vi "MLS ident.vi"() -> ()   [LabVIEW 2015]
uses:
  <vilib>/FPGAPlugInAG/myRIO-1900/niLvFpga_Open_myRIO-1900.vi
  <vilib>/rvi/interface/common/dynamic/niFpgaDynamicAddResources.vi
  <vilib>/Utility/file.llb/Write Delimited Spreadsheet (I64).vi
  <vilib>/Utility/file.llb/Write Delimited Spreadsheet (DBL).vi
  <vilib>/Utility/error.llb/Error Cluster From Error Code.vi
  <vilib>/rvi/errors/niLvFpgaAdjustHostInterfaceError.vi
  <vilib>/FPGAPlugInAG/Dynamic/niLvFpga_Close_Dynamic.vi
  <vilib>/rvi/interface/nirviOpenFPGA/nirviOpenFPGA.xnode
  FPGA Bitfiles/ACC20115_FPGATarget_CurrentControlle_Dt5vFgOzYtY.lvbitx
  Current Controller.vi
  <vilib>/rvi/interface/nirviReadWriteControl/nirviReadWriteControl.xnode
  <vilib>/rvi/interface/nirviCloseFPGA/nirviCloseFPGA.xnode
  <vilib>/Analysis/NI_AALBase.lvlib
  NiFpgaLv.dll
  <vilib>/rvi/interface/Simulation/niFpgaSimulationCallBeginRW.vi
panel:
  out "error out":errorcluster
  in  "Stop":bool
  in  "Tab Control":enum32{"Monitor"}(tab)
  out "MLS":dbl[](graph)
  out "Sensor":dbl(graph)
  out "FPGA Status":bool
  out "Uniform White Noise":dbl[](graph)
  out "ms":u32
  in  "samples":i64=1
  out "Sampling Frequency":dbl(graph)
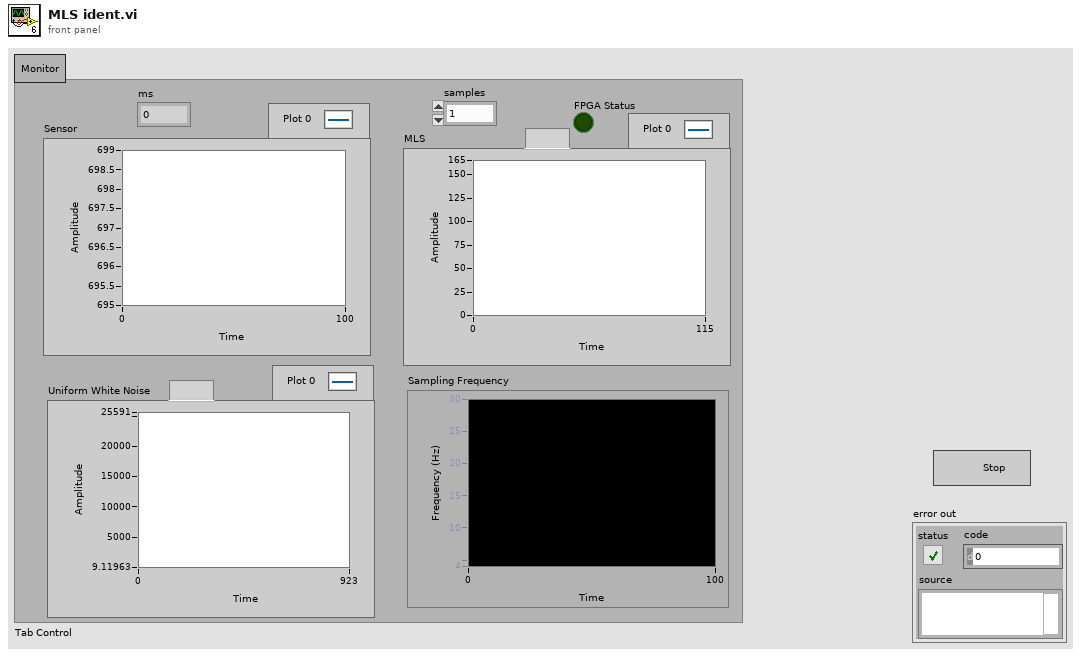
[diagram p1: front panel]
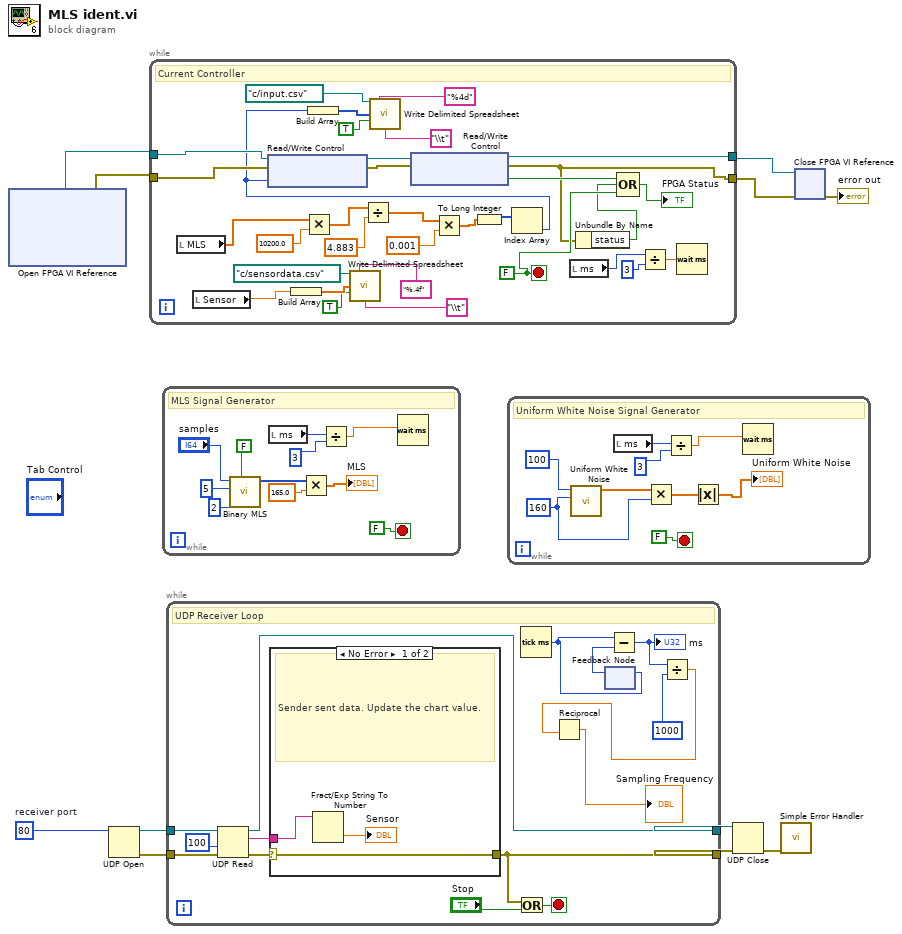
[diagram p0: block diagram]
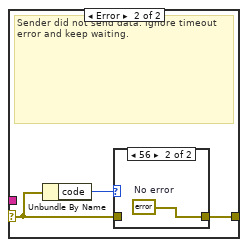
[diagram p2: hidden frame]
diagram:
  w2 = u16 80  # receiver port
  n1 = xnode "Open FPGA VI Reference"() -> ("FPGA VI Reference Out"=w11:refnum<k20>, "error out"=w10:errorcluster)  [unwired: 2 in]
  n2 = UDP Open(11:w2) -> (port=w3:refnum<k16>, 0:w4:errorcluster)  [unwired: 4 in, 1 out]
  n3 = while {
    tunnel: w11 -> [w44]
    tunnel: w10 -> [w43]
    tunnel: [w33] -> w9
    tunnel: [w29] -> w8
    stop <- w32 stop-if-true
    w32 = FALSE
    # "Current Controller"
    n4 = local read "MLS"() -> (w38:dbl[])
    n5 = local read "Sensor"() -> (w16:dbl)
    n6 = Build Array(w16) -> (w17:dbl[])
    n7 = Multiply(x=w38, y=10200.0) -> (x*y=w39:dbl[])
    n8 = call-poly <vilib>:"Write Delimited Spreadsheet.vi"("file path (dialog if empty)"=path "c:/sensordata.csv", "format (%.3f)"="%.4f", "1D data"=w17, "append to file? (F)"=TRUE, "delimiter (\\t)"="\\t" ("delimiter (\\t)")) -> ()  [unwired: 9 in, 2 out]
    n9 = Divide(x=w39, y=4.883) -> (x/y=w41:dbl[])
    n10 = Multiply(x=w41, y=0.001) -> (x*y=w37:dbl[])
    n11 = To Long Integer(number=w37) -> (32bit integer=w24:i32[])
    n12 = Index Array(array=w24) -> (element=w23:i32)  [unwired: 1 in]
    n13 = xnode "Read/Write Control"("FPGA VI Reference In"=w44, "error in"=w43, "DAC Inlet Valve"=w23) -> ("FPGA VI Reference Out"=w35:refnum<k20>, "error out"=w34:errorcluster)
    n14 = Build Array(w23) -> (w22:i32[])
    n15 = call-poly <vilib>:"Write Delimited Spreadsheet.vi"("file path (dialog if empty)"=path "c:/input.csv", "format (%d)"="%4d", "1D data"=w22, "append to file? (F)"=TRUE, "delimiter (\\t)"="\\t" ("delimiter (\\t)")) -> ()  [unwired: 9 in, 2 out]
    n16 = xnode "Read/Write Control"("FPGA VI Reference In"=w35, "error in"=w34) -> ("FPGA VI Reference Out"=w33:refnum<k20>, "error out"=w29:errorcluster, "Inlet Overflow?"=w30:bool)
    n17 = local read "ms"() -> (w28:u32)
    n18 = Unbundle By Name(w29) -> ("status"=w31:bool)
    n19 = Compound Arithmetic op=OR(w30, w31, w32) -> (→"FPGA Status":bool)
    n20 = Divide(x=w28, y=u32 3) -> (x/y=w26:dbl)
    n21 = Wait (ms)(milliseconds to wait=w26) -> ()  [unwired: 1 out]
  }
  n22 = while {
    stop <- FALSE stop-if-true
    # "MLS Signal Generator"
    n23 = call <vilib>:"Binary MLS.vi"("initialize?"=FALSE, "seed"=i64 2, "polynomial order"=5, "samples"="samples") -> ("mls sequence"=w52:u8[])  [unwired: 6 in, 1 out]
    n24 = local read "ms"() -> (w50:u32)
    n25 = Multiply(x=w52, y=165.0 ("amplitude")) -> (x*y=→"MLS":dbl[])
    n26 = Divide(x=w50, y=u32 3) -> (x/y=w48:dbl)
    n27 = Wait (ms)(milliseconds to wait=w48) -> ()  [unwired: 1 out]
  }
  n28 = while {
    tunnel: w3 -> [w70]
    tunnel: [w62] -> w7
    tunnel: w4 -> [w67]
    tunnel: [w63] -> w5
    stop <- w68 stop-if-true
    # "UDP Receiver Loop"
    n29 = UDP Read(connection ID=w70, timeout ms (25000)=100, 8:w67) -> (data out=w65:string, error out=w64:errorcluster, 3:w62:refnum<k16>)  [unwired: 3 out]
    n30 = case shown="No Error" w64 {
      selector: w64 -> [w71 w75]
      tunnel: w65 -> [w73 _]
      tunnel: [w71 w74] -> w63
      frame No Error {
        # "Sender sent data. Update the chart value."
        n31 = Fract/Exp String To Number(string=w73) -> (number=→"Sensor":dbl)  [unwired: 3 in, 1 out]
      }
      frame Error {
        # "Sender did not send data. Ignore timeout error and keep waiting."
        n32 = Unbundle By Name(w75) -> ("code"=w76:i32)
        n33 = case shown="56" w76 {
          tunnel: w75 -> [w77 _]
          tunnel: [w77 w78] -> w74
          frame Default {
          }
          frame 56 {
            w78 = errorcluster {"status"=FALSE, "code"=0, "source"=""}  # No error
          }
        }
      }
    }
    n34 = Or(x=w63, y="Stop") -> (x .or. y?=w68:bool)
    n35 = Tick Count (ms)() -> (millisecond timer value=w61:u32)
    n36 = feedback-in #1(w61) -> ()
    n37 = feedback #1() -> (w60:u32)  [unwired: 1 in]
    n38 = Subtract(x=w61, y=w60) -> (x-y=w58:u32)
    "ms" <- w58
    n39 = Divide(x=w58, y=u32 1000) -> (x/y=w57:dbl)
    n40 = Reciprocal(x=w57) -> (1/x=→"Sampling Frequency":dbl)
  }
  n41 = while {
    stop <- FALSE stop-if-true
    w81 = 160 ("polynomial order")
    # "Uniform White Noise Signal Generator"
    n42 = call <vilib>:"Uniform White Noise.vi"("amplitude"=w81, "samples"=i64 100) -> ("uniform white noise"=w83:dbl[])  [unwired: 8 in, 1 out]
    n43 = local read "ms"() -> (w86:u32)
    n44 = Multiply(x=w83, y=w81) -> (x*y=w80:dbl[])
    n45 = Divide(x=w86, y=u32 3) -> (x/y=w84:dbl)
    n46 = Absolute Value(x=w80) -> (abs(x)=→"Uniform White Noise":dbl[])
    n47 = Wait (ms)(milliseconds to wait=w84) -> ()  [unwired: 1 out]
  }
  n48 = UDP Close(connection ID=w7, 8:w5) -> (error out=w6:errorcluster)  [unwired: 1 out]
  n49 = call <vilib>:"Simple Error Handler.vi"("error in (no error)"=w6) -> ()  [unwired: 1 in, 8 out]
  n50 = xnode "Close FPGA VI Reference"("FPGA VI Reference In"=w9, "error in"=w8) -> ("error out"=→"error out":errorcluster)
